vi "Read Report File.vi"(0 "Display State In":T1={"ImageSource"=enum."Camera", "IMAQdx Cam"=refnum, "WorkDir"=path "", "Image Name Prefix"="", "ROI"={"Global Rectangle"=[], "Contours"=[]}, "BG Image"=refnum, "Display Image"=refnum, "Display settings"={"Min. Thresh."=0.0, "X"=0.0, "Y"=0.0, "ShowLineout"=FALSE, "ScaleParts"=10, "ShowLegende"=FALSE, "Target Cross"=FALSE, "Centroid Cross"=FALSE, "Target color"=16777226, "Centroid color"=16711680, "calibr. mm/px"=0.0}, "Mask image"=refnum, "ConfigDir"=path "", "Display ref"=refnum, "Saved ROIs"=[], "Selected ROI"="", "Analyze Objects"=[], "Analysis Params"=variant, "Analysis Results"=variant, "Overlays?"=[], "Ref Palette type"=refnum, "Time in Filename?"=TRUE, "Save Report?"=TRUE, "Appl Params"=variant, "Show ZoomBtn?"=TRUE, "Image file"=path "", "SubstractBG?"=TRUE, "Centroid"={"X Centroid"=0.0, "Y Centroid"=0.0}, "Image In"=refnum} {"Centroid"."Y Centroid" format="%.2f"; "Centroid"."X Centroid" format="%.2f"; "ROI"."Contours"."Type" items=["No Selection", "Point", "Line", "Rectangle", "Oval", "Polygon", "Freehand Region", "Annulus", "Unused2", "Unused3", "Broken Line", "Freehand Line", "Rotated Rectangle"]}, 5 "Path":path, 9 "Container State":T7, 11 "error in (no error)":errorcluster) -> (4 "Display State Out":T1={"ImageSource"=enum."Camera", "IMAQdx Cam"=refnum, "WorkDir"=path "", "Image Name Prefix"="", "ROI"={"Global Rectangle"=[], "Contours"=[]}, "BG Image"=refnum, "Display Image"=refnum, "Display settings"={"Min. Thresh."=0.0, "X"=0.0, "Y"=0.0, "ShowLineout"=FALSE, "ScaleParts"=10, "ShowLegende"=FALSE, "Target Cross"=FALSE, "Centroid Cross"=FALSE, "Target color"=16777226, "Centroid color"=16711680, "calibr. mm/px"=0.0}, "Mask image"=refnum, "ConfigDir"=path "", "Display ref"=refnum, "Saved ROIs"=[], "Selected ROI"="", "Analyze Objects"=[], "Analysis Params"=variant, "Analysis Results"=variant, "Overlays?"=[], "Ref Palette type"=refnum, "Time in Filename?"=TRUE, "Save Report?"=TRUE, "Appl Params"=variant, "Show ZoomBtn?"=TRUE, "Image file"=path "", "SubstractBG?"=TRUE, "Centroid"={"X Centroid"=0.0, "Y Centroid"=0.0}, "Image In"=refnum} {"Centroid"."Y Centroid" format="%.2f"; "Centroid"."X Centroid" format="%.2f"; "ROI"."Contours"."Type" items=["No Selection", "Point", "Line", "Rectangle", "Oval", "Polygon", "Freehand Region", "Annulus", "Unused2", "Unused3", "Broken Line", "Freehand Line", "Rotated Rectangle"]}, 15 "error out":errorcluster)   [LabVIEW 2014, in "POLARIS IMAQ Display.xctl"]
uses:
  POLARIS IMAQ Display.xctl
  <vilib>/_xctls/Container State.ctl
  State.ctl
  IMAQdx Cam/IMAQdx Cam.lvclass
  Properties/ImageSource.ctl
  <vilib>/vision/Image Controls.llb/IMAQ Image.ctl
  DisplaySettings.ctl
  Named ROI.ctl
  Analyze Classes/Analyze BaseClass/Analyze BaseClass.lvclass
  Palette.ctl
  Utility/POLARIS Vision utility.lvlib
  <vilib>/Utility/config.llb/NI_LVConfig.lvlib
  <vilib>/_xctls/XControlSupport.lvlib
panel:
  # "Add Controls & Indicators that form the parameters of the method here. Hook them to the connector pane. Do not delete the controls & indicators that are already hooked to the connector pane.\n \nTo setup the parameters  for this method, right click on this item in the Project Tree & select \"Configure Method...\"."
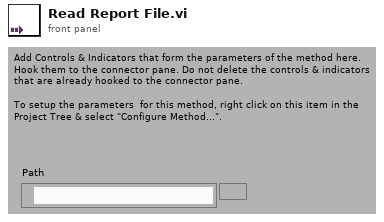
[diagram p1: front panel]
types:
  T1 = typedef "POLARIS IMAQ Display.xctl/State.ctl" = cluster{"ImageSource":T2, "IMAQdx Cam":refnum<class "IMAQdx Cam.lvclass">, "WorkDir":path, "Image Name Prefix":string, "ROI":T3, "BG Image":T4, "Display Image":T4, "Display settings":T5, "Mask image":T4, "ConfigDir":path, "Display ref":refnum<vi>, "Saved ROIs":T6[], "Selected ROI":string, "Analyze Objects":refnum<class "Analyze BaseClass.lvclass">[], "Analysis Params":variant, "Analysis Results":variant, "Overlays?":bool[], "Ref Palette type":refnum<vi>, "Time in Filename?":bool, "Save Report?":bool, "Appl Params":variant, "Show ZoomBtn?":bool, "Image file":path, "SubstractBG?":bool, "Centroid":cluster{"X Centroid":sgl, "Y Centroid":sgl}, "Image In":T4}
  T2 = typedef "POLARIS IMAQ Display.xctl/ImageSource.ctl" = enum16{"Camera", "File"}
  T3 = typedef "ROI Descriptor" = cluster{"Global Rectangle":i32[], "Contours":cluster{"ID":enum32{"External", "Internal"}, "Type":u32, "Coordinates":i32[]}[]}
  T4 = typedef "IMAQ Image.ctl" = refnum<image>
  T5 = typedef "POLARIS IMAQ Display.xctl/DisplaySettings.ctl" = cluster{"Min. Thresh.":sgl, "X":dbl, "Y":dbl, "ShowLineout":bool, "ScaleParts":i32, "ShowLegende":bool, "Target Cross":bool, "Centroid Cross":bool, "Target color":u32, "Centroid color":u32, "calibr. mm/px":sgl}
  T6 = typedef "POLARIS IMAQ Display.xctl/Named ROI.ctl" = cluster{"ROI":cluster{"Global Rectangle":i32[], "Contours":cluster{"Contour Type":u32, "ROI Type":u32, "Points":i32[]}[]}, "Name":string}
  T7 = typedef "XControlSupport.lvlib/Container State.ctl" = cluster{"Indicator?":bool, "Run Mode?":bool, " Refnum":refnum<vi>}
  T8 = typedef "NI_LVConfig.lvlib/Config Data RefNum.ctl" = refnum<k1>
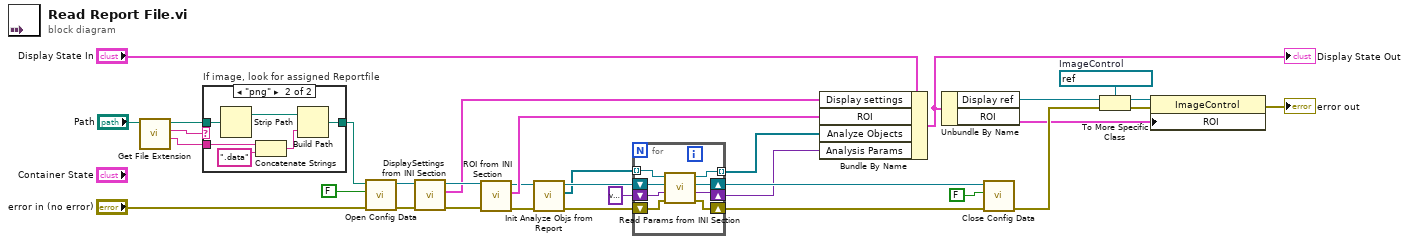
[diagram p0: block diagram]
diagram:
  w10 = refnum<vi> refnum  # ImageControl
  n1 = call <vilib>:"Get File Extension.vi"("file"="Path") -> ("filename without extension"=w29:string, "lowercase file extension"=w31:string, "dup file"=w30:path)  [unwired: 7 in, 1 out]
  n2 = case "If image, look for assigned Reportfile" shown="\"png\"" w31 {
    tunnel: w30 -> [w34 w40]
    tunnel: [w34 w39] -> w28
    tunnel: w29 -> [_ w37]
    frame "data", Default {
    }
    frame "png" {
      n3 = Strip Path(path=w40) -> (stripped path=w38:path)  [unwired: 1 out]
      n4 = Concatenate Strings(w37, ".data" ("string")) -> (w35:string)
      n5 = Build Path(base path=w38, name or relative path=w35) -> (appended path=w39:path)
    }
  }
  n6 = call <vilib>:"Open Config Data.vi"("error in (no error)"="error in (no error)", "create file if necessary (T)"=FALSE, "configuration file path"=w28) -> ("error out"=w24:errorcluster, "refnum"=w25:T8)  [unwired: 6 in, 1 out]
  n7 = call "DisplaySettings from INI Section.vi"("error in (no error)"=w24, "refnum in"=w25) -> ("error out"=w22:errorcluster, "Display settings"=w21:T5, "refnum out"=w23:T8)  [unwired: 7 in]
  n8 = call "ROI from INI Section.vi"("error in (no error)"=w22, "refnum in"=w23) -> ("error out"=w7:errorcluster, "ROI"=w15:T3, "refnum out"=w9:T8)  [unwired: 7 in]
  n9 = call "Init Analyze Objs from Report.vi"("error in (no error)"=w7, "refnum in"=w9) -> ("error out"=w6:errorcluster, "Selected Objs"=w5:refnum<class "Analyze BaseClass.lvclass">[], "refnum out"=w8:T8)  [unwired: 6 in, 1 out]
  n10 = for {
    tunnel: w5 -> [w47] mode=indexing
    shift-right: [w45] -> w12
    shift-left: w6 -> [w46]
    shift-right: [w44] -> w11
    shift-left: w8 -> [w48]
    shift-right: [w42] -> w1
    shift-left: variant ("Parameters In") -> [w43]
    tunnel: [w41] -> w2 mode=indexing
    n11 = call-dynamic "Read Params from INI Section.vi"("error in (no error)"=w46, "Parameters In"=w43, "Refnum in"=w48, "Analyze BaseClass in"=w47) -> ("error out"=w45:errorcluster, "Parameters Out"=w42:variant, "Refnum out"=w44:T8, "Analyze BaseClass out"=w41:refnum<class "Analyze BaseClass.lvclass">)  [unwired: 4 in]
  }
  n12 = Bundle By Name(cluster="Display State In", "Display settings"=w21, "ROI"=w15, "Analyze Objects"=w2, "Analysis Params"=w1) -> (w4:T1)
  "Display State Out" <- w4
  n13 = Unbundle By Name(w4) -> ("Display ref"=w19:refnum<vi>, "ROI"=w3:T3)
  n14 = call <vilib>:"Close Config Data.vi"("error in (no error)"=w12, "write file if changed (T)"=FALSE, "refnum"=w11) -> ("error out"=w17:errorcluster)  [unwired: 7 in, 1 out]
  n15 = To More Specific Class(target class=w10, reference=w19, error in=w17) -> (specific class reference=w18:refnum<vi>, error out=w16:errorcluster)
  n16 = property class="ImageControl"(reference=w18, error in=w16, "ROI"=w3) -> (error out=→"error out":errorcluster)  [unwired: 1 out]
